vi "Set Alias Endpoint.vi"(8 "error in":errorcluster, 9 "new endpoint":T1, 10 "alias":string, 11 "endpoint aliases in":T2 format="%.0x") -> (0 "error out":errorcluster, 3 "endpoint aliases out":T2 format="%.0x")   [LabVIEW 2020, in "Routing and Faulting Scripting.lvlib"]
doc: "Sets the endpoint for an existing alias."
uses:
  Routing and Faulting Scripting.lvlib
  <vilib>/NI VeriStand/Custom Device API/Custom Device Item Ref.ctl
  Shared/Alias Endpoint.ctl
  <vilib>/NI VeriStand/Custom Device API/Set Item Property (String).vi
  <vilib>/NI VeriStand/Custom Device API/Custom Device API.lvlib
  Dependencies.llb/Routing and Faulting Shared.lvlib
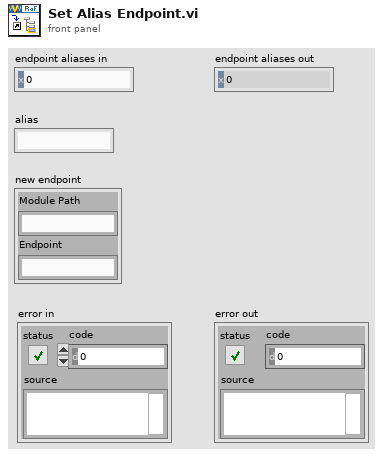
[diagram p1: front panel]
types:
  T1 = typedef "Routing and Faulting Shared.lvlib/Alias Endpoint.ctl" = cluster{"Module Path":string, "Endpoint":string}
  T2 = typedef "Custom Device API.lvlib/Custom Device Item Ref.ctl" = u64
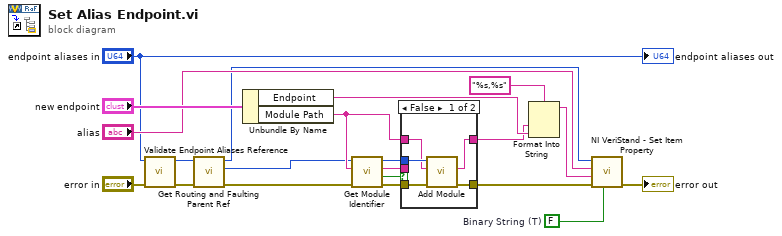
[diagram p0: block diagram]
diagram:
  w19 = FALSE  # Binary String (T)
  n1 = call "Validate Endpoint Aliases Reference.vi"("error in"="error in", "endpoint aliases in"="endpoint aliases in") -> ("error out"=w2:errorcluster, "endpoint aliases out"=w1:T2)  [unwired: 8 in]
  n2 = call "Get Routing and Faulting Parent Ref.vi"("error in"=w2, "routing and faulting child in"=w1) -> ("error out"=w15:errorcluster, "routing and faulting"=w3:T2, "routing and faulting child out"=w8:T2)  [unwired: 7 in]
  n3 = Unbundle By Name("new endpoint") -> ("Endpoint"=w18:string, "Module Path"=w7:string)
  n4 = call "Get Module Identifier.vi"("error in"=w15, "module path"=w7, "routing and faulting in"=w3) -> ("error out"=w12:errorcluster, "found?"=w13:bool, "module identifier"=w14:string, "routing and faulting out"=w11:T2)  [unwired: 5 in]
  n5 = case shown="False" w13 {
    tunnel: w11 -> [w26 _]
    tunnel: w7 -> [w25 _]
    tunnel: w12 -> [w24 w27]
    tunnel: [w23 w27] -> w16
    tunnel: w14 -> [_ w28]
    tunnel: [w22 w28] -> w17
    frame False {
      n6 = call "Add Module.vi"("error in"=w24, "module path"=w25, "routing and faulting in"=w26) -> ("error out"=w23:errorcluster, "unique module identifier"=w22:string)  [unwired: 6 in, 1 out]
    }
    frame True {
    }
  }
  n7 = Format Into String(format string="%s,%s", w17, w18) -> (resulting string=w9:string)  [unwired: 2 in, 1 out]
  n8 = call-poly <vilib>:"NI VeriStand - Set Item Property.vi"("Binary String (T)"=w19, "error in (no error)"=w16, "Value"=w9, "Property Name"="alias", "Item Ref in"=w8) -> ("error out"=→"error out":errorcluster)  [unwired: 4 in, 2 out]
  "endpoint aliases out" <- "endpoint aliases in"
